vi "Introspection Core.vi"(8 "error in (no error)":errorcluster, 11 "IVI_Scope in":refnum<class "IVI_Scope.lvclass">) -> (0 "error out":errorcluster, 2 "CS++Messages":refnum<class "Message.lvclass">[](array[class]), 3 "IVI_Scope out":refnum<class "IVI_Scope.lvclass">)   [LabVIEW 2014, in "IVI_Scope.lvlib" / "IVI_Scope.lvclass"]
doc: "This vi delivers a list with all messages this actor reacts to. \n\nNote that all inherited classes have to overwrite it."
uses:
  IVI_Scope.lvclass
  CSPP_DeviceBase/CS++Scope/CS++Scope.lvclass
  <vilib>/ActorFramework/Message/Message.lvclass
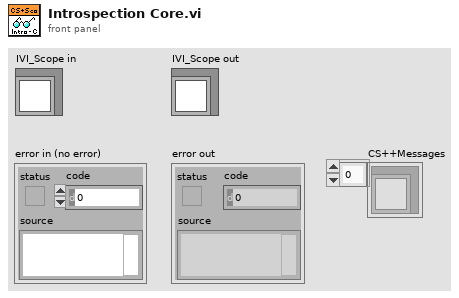
[diagram p1: front panel]
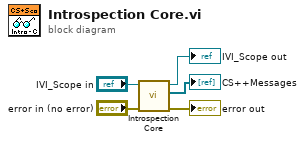
[diagram p0: block diagram]
diagram:
  n1 = call-parent "Introspection Core.vi"("error in (no error)"="error in (no error)", "CS++Scope in"="IVI_Scope in") -> ("error out"=→"error out":errorcluster, "CS++Messages"=→"CS++Messages":refnum<class "Message.lvclass">[], "CS++Scope out"=→"IVI_Scope out":refnum<class "IVI_Scope.lvclass">)  [unwired: 7 in]
